vi "Receive Event.vi"(8 "Error In":errorcluster, 9 "Event Data":refnum<class "Event Data.lvclass">, 10 "Event Name":string, 11 "Chat Window Model In":refnum<class "Chat Window Model.lvclass">) -> (0 "Error Out":errorcluster, 3 "Chat Window Model Out":refnum<class "Chat Window Model.lvclass">)   [LabVIEW 2020, in "Chat Window Model.lvlib" / "Chat Window Model.lvclass"]
uses:
  Chat Window Model.lvclass
  C:/Program Files/National Instruments/LabVIEW 2020/vi.lib/ActorFramework/Actor/Actor.lvclass
  SubPanel-Actor-Framework-master/Event-Source-Actor/Source/Template Source/Event Data/Event Data.lvclass
  <vilib>/ActorFramework/Actor/Actor.lvclass/Actor.ctl
  <vilib>/ActorFramework/Message Enqueuer/Message Enqueuer.lvclass/Message Enqueuer.ctl
  Event-Source-Actor/Data Interface/VI Info Data/VI Info Data.lvclass
  Chat Window Model Messages/New Panel Launched Msg/New Panel Launched Msg.lvclass/New Panel Launched Msg.ctl
  Event-Source-Actor/Data Interface/Status Data/Status Data.lvclass
  Chat Window Model Messages/User Updated Status Msg/User Updated Status Msg.lvclass/User Updated Status Msg.ctl
  Event-Source-Actor/Data Interface/Message Data/Message Data.lvclass
  Chat Window Model Messages/Forward Direct Message Msg/Forward Direct Message Msg.lvclass/Forward Direct Message Msg.ctl
  <vilib>/ActorFramework/Message Enqueuer/Init from Existing Queue.vi
  <vilib>/ActorFramework/Message Enqueuer/Enqueue.vi
  Chat Window Model Messages/New Panel Launched Msg/New Panel Launched Msg.lvclass
  C:/Program Files/National Instruments/LabVIEW 2020/vi.lib/ActorFramework/Message/Message.lvclass
  Chat Window Model Messages/User Updated Status Msg/User Updated Status Msg.lvclass
  Chat Window Model Messages/Forward Direct Message Msg/Forward Direct Message Msg.lvclass
  <vilib>/ActorFramework/Message Priority Queue/Priority Enqueue.vi
  <vilib>/ActorFramework/Message Enqueuer/Message Enqueuer.lvclass
  Chat Window Model.lvclass/Chat Window Model.ctl
  <vilib>/ActorFramework/Actor/Actor.lvclass
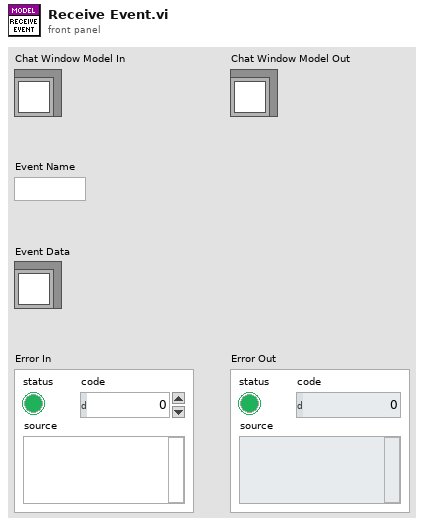
[diagram p1: front panel]
types:
  T1 = typedef "Message Control.ctl" = cluster{"From":string, "To":string, "Message":string}
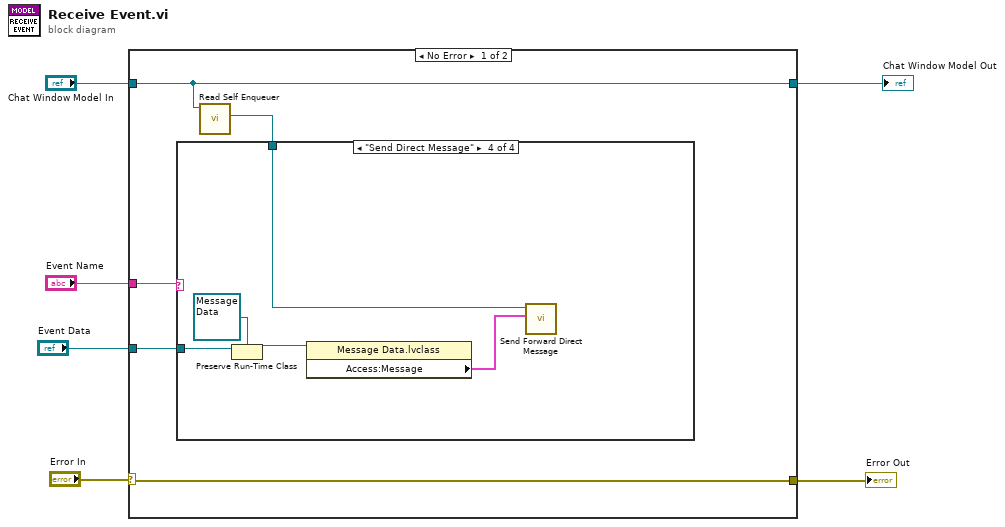
[diagram p0: block diagram]
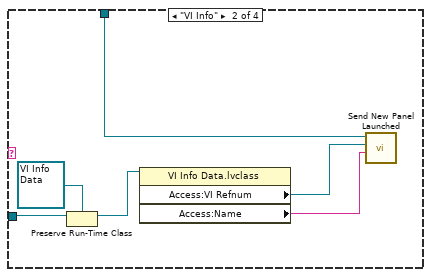
[diagram p3: hidden frame]
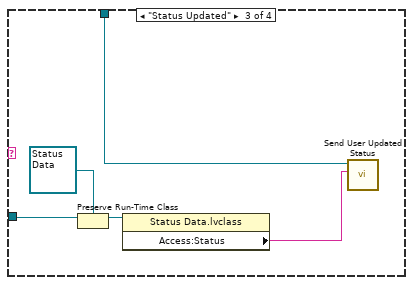
[diagram p4: hidden frame]
diagram:
  n1 = case shown="No Error" "Error In" {
    selector: "Error In" -> [w11 w28]
    tunnel: [w11 w28] -> w5
    tunnel: "Chat Window Model In" -> [w9 w29]
    tunnel: [w9 w29] -> w3
    tunnel: "Event Name" -> [w10 _]
    tunnel: "Event Data" -> [w7 _]
    frame No Error {
      n2 = call <vilib>:"Read Self Enqueuer.vi"("Actor"=w9) -> ("Self Enqueuer"=w8:refnum<class "Message Enqueuer.lvclass">)  [unwired: 10 in]
      n3 = case shown="\"Send Direct Message\"" w10 {
        tunnel: w8 -> [_ w17 w19 w27]
        tunnel: w7 -> [_ w16 w21 w25]
        frame "False", Default {
        }
        frame "VI Info" {
          n4 = Preserve Run-Time Class(object in=w16, 2:refnum<class "VI Info Data.lvclass"> refnum ("VI Info Data.lvclass")) -> (object out=w14:refnum<class "VI Info Data.lvclass">)  [unwired: 1 in, 1 out]
          n5 = property class="VI Info Data.lvclass"(reference=w14) -> ("Access:VI Refnum"=w13:refnum<vi>, "Access:Name"=w12:string)  [unwired: 1 in, 2 out]
          n6 = call "Send New Panel Launched.vi"("Name"=w12, "VI Refnum"=w13, "Message Enqueuer in"=w17) -> ()  [unwired: 7 in, 2 out]
        }
        frame "Status Updated" {
          n7 = Preserve Run-Time Class(object in=w21, 2:refnum<class "Status Data.lvclass"> refnum ("Status Data.lvclass")) -> (object out=w20:refnum<class "Status Data.lvclass">)  [unwired: 1 in, 1 out]
          n8 = property class="Status Data.lvclass"(reference=w20) -> ("Access:Status"=w18:string)  [unwired: 1 in, 2 out]
          n9 = call "Send User Updated Status.vi"("Status"=w18, "Message Enqueuer in"=w19) -> ()  [unwired: 8 in, 2 out]
        }
        frame "Send Direct Message" {
          n10 = Preserve Run-Time Class(object in=w25, 2:refnum<class "Message Data.lvclass"> refnum ("Message Data.lvclass")) -> (object out=w24:refnum<class "Message Data.lvclass">)  [unwired: 1 in, 1 out]
          n11 = property class="Message Data.lvclass"(reference=w24) -> ("Access:Message"=w23:T1)  [unwired: 1 in, 2 out]
          n12 = call "Send Forward Direct Message.vi"("Message"=w23, "Message Enqueuer in"=w27) -> ()  [unwired: 8 in, 2 out]
        }
      }
    }
    frame Error {
    }
  }
  "Chat Window Model Out" <- w3
  "Error Out" <- w5
